vi "Disconnect.vi"(8 "error in":errorcluster, 11 "69X_79X in":refnum<class "7976A.lvclass">) -> (0 "error out":errorcluster, 3 "69X_79X out":refnum<class "7976A.lvclass">)   [LabVIEW 2019, in "7976A.lvlib" / "7976A.lvclass"]
uses:
  Library/7976A.lvclass
  Library/7976A.lvclass/7976A.ctl
  <instrlib>/Agilent N7976A/Agilent N7976A.lvlib
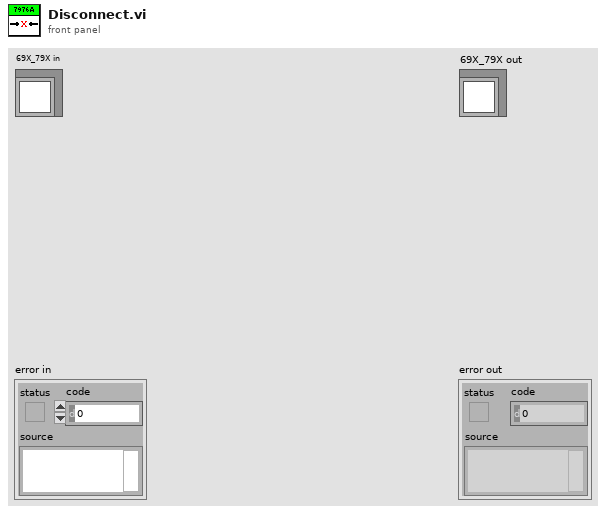
[diagram p1: front panel]
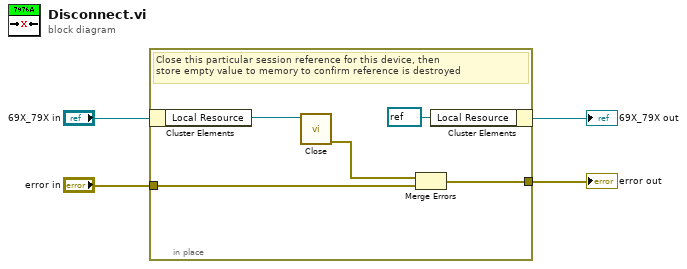
[diagram p0: block diagram]
diagram:
  n1 = in-place {
    in-place-border: "error in" -> [w9]
    in-place-border: [w8] -> w2
    # "Close this particular session reference for this device, then\nstore empty value to memory to confirm reference is destroyed"
    n2 = in-place-cluster #1("69X_79X in") -> ("Local Resource"=w6:refnum<visa-resource-name>)
    n3 = call <instrlib>:"Close.vi"("VISA resource name"=w6) -> ("error out"=w5:errorcluster)  [unwired: 10 in]
    n4 = Merge Errors(w5, w9) -> (w8:errorcluster)
    n5 = in-place-cluster #1("Local Resource"=refnum<visa-resource-name> refnum) -> (→"69X_79X out":refnum<class "7976A.lvclass">)
  }
  "error out" <- w2
